vi "is invalid.vi"(11 "stream publisher in":refnum<class "data bus stream subscriber.lvclass">) -> (2 "invalid?":bool, 3 "stream publisher out":refnum<class "data bus stream subscriber.lvclass">)   [LabVIEW 2013, in "data bus stream subscriber.lvclass"]
uses:
  data bus stream subscriber.lvclass
  data bus stream subscriber.lvclass/data bus stream subscriber.ctl
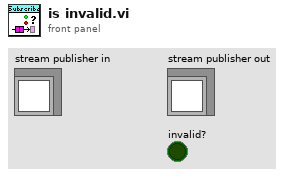
[diagram p1: front panel]
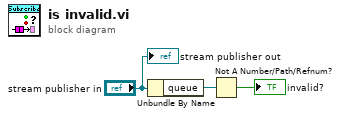
[diagram p0: block diagram]
diagram:
  n1 = Unbundle By Name("stream publisher in") -> ("queue"=w2:refnum<queue>)
  n2 = Not A Number/Path/Refnum?(number/path/refnum=w2) -> (NaN/Path/Refnum?=→"invalid?":bool)
  "stream publisher out" <- "stream publisher in"
